vi "get_image.vi"(8 "error in":errorcluster, 9 "height":i32=512, 10 "width":i32=240) -> (0 "error out":errorcluster, 1 "data":u16[][](array[numeric]), 2 "获取单帧图像返回值":i32, 3 "Image":T1(plugin-control), 4 "Intensity Graph":u16[][](graph))   [LabVIEW 2016]
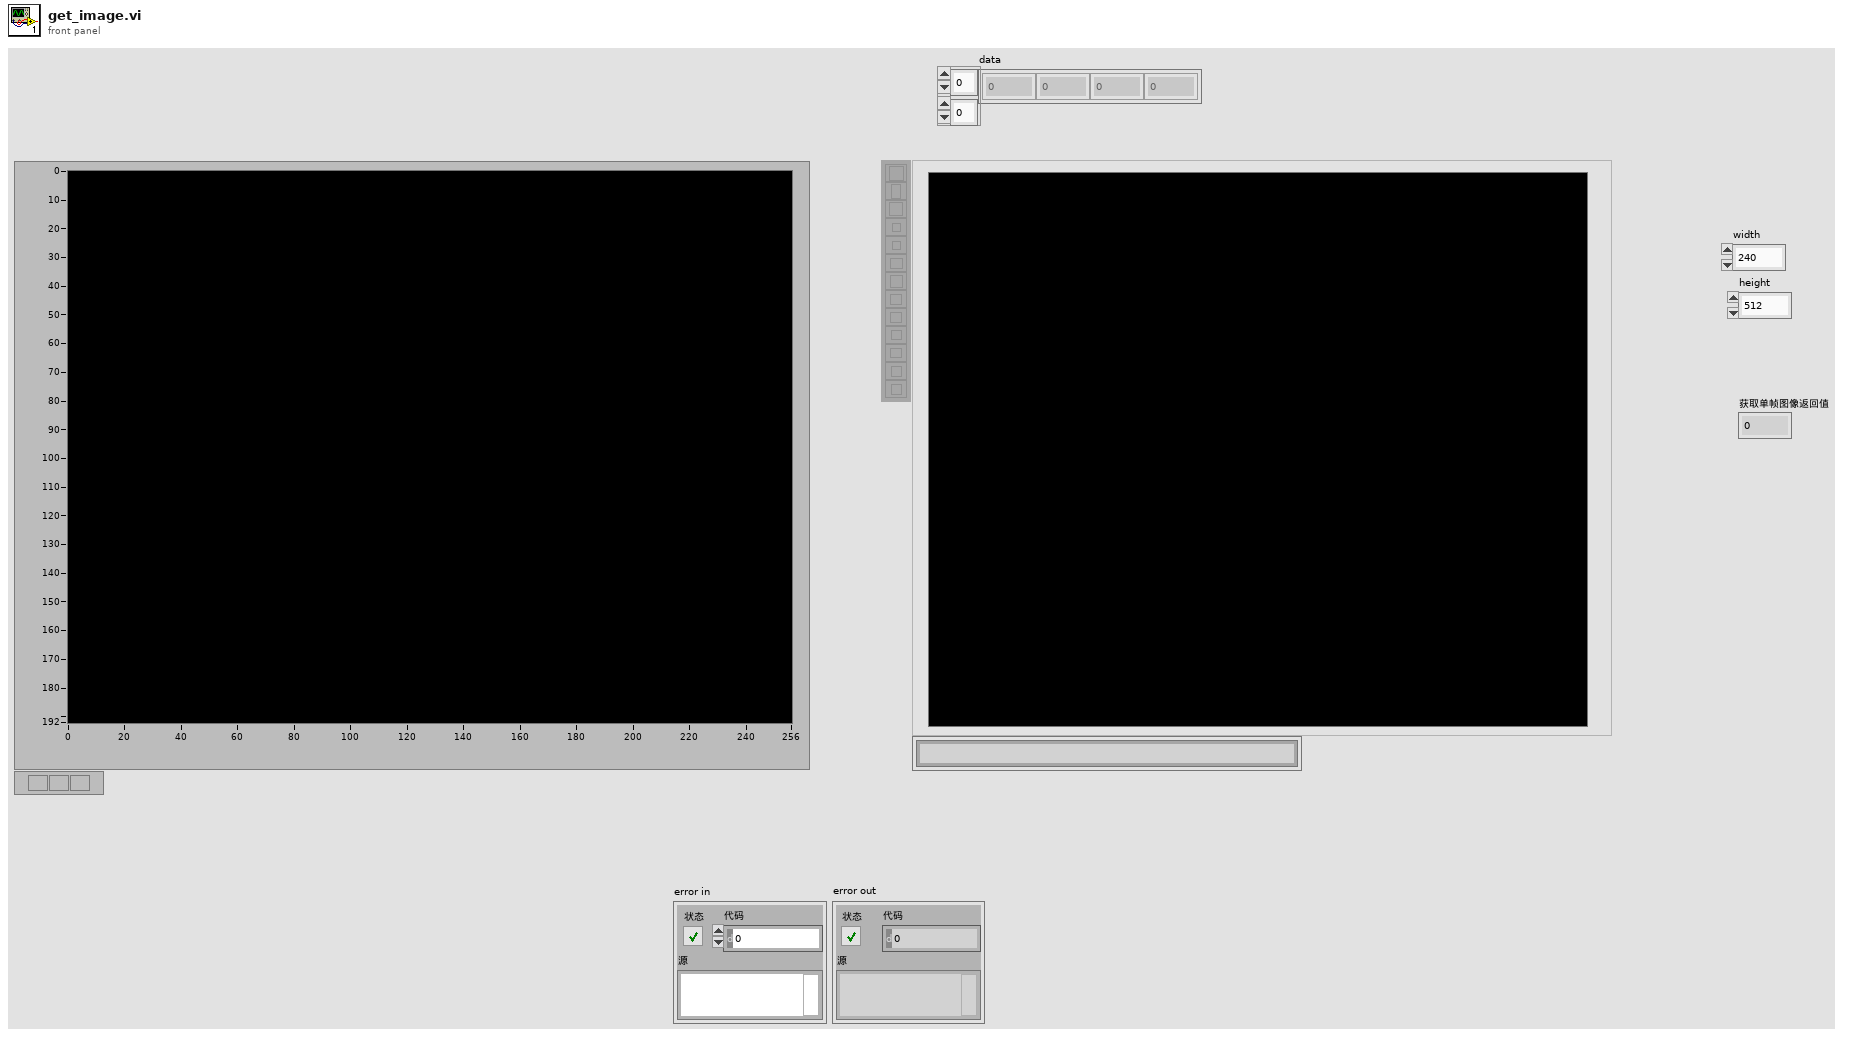
[diagram p1: front panel]
types:
  T1 = typedef "IMAQ Image.ctl" = refnum<image>
  T2 = typedef "Image Type" = u32
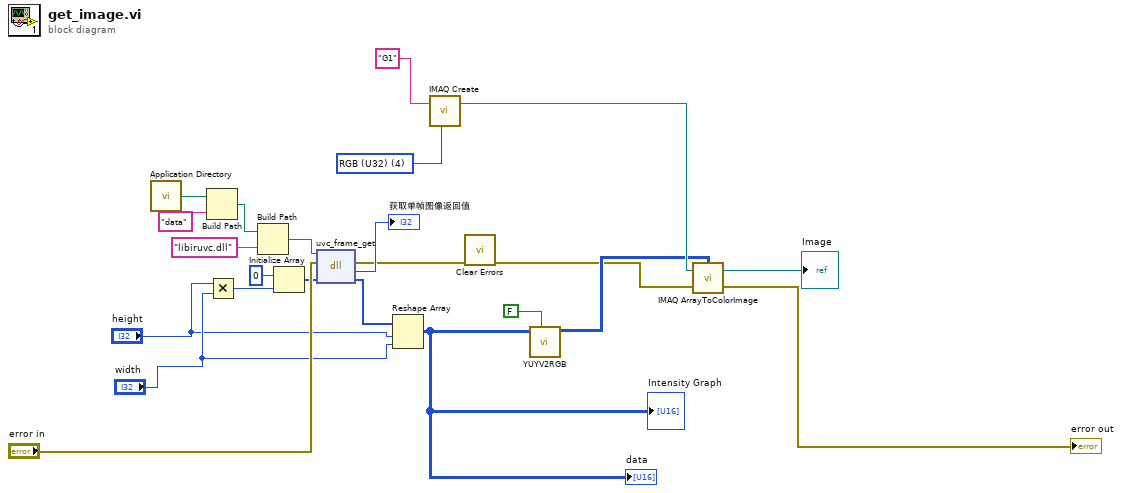
[diagram p0: block diagram]
diagram:
  w23 = T2 4 items=["Grayscale (U8)", "Grayscale (I16)", "Grayscale (SGL)", "Complex (CSG)", "RGB (U32)", "HSL (U32)", "RGB (U64)", "Grayscale (U16)"] ("Image Type")
  n1 = call <vilib>:"Application Directory.vi"() -> ("Application Directory"=w11:path)
  n2 = Build Path(base path=w11, name or relative path="data") -> (appended path=w9:path)
  n3 = Multiply(x="height", y="width") -> (x*y=w14:i32)
  n4 = Build Path(base path=w9, name or relative path="libiruvc.dll") -> (appended path=w15:path)
  n5 = Initialize Array(u16 0, w14) -> (w12:u16[])
  n6 = dll-call lib="D:/libiruvc_0.3.3/windows/x64/dll/libiruvc.dll" fn="uvc_frame_get"(path in=w15, error in="error in", "data"=w12) -> (error out=w6:errorcluster, "return type"=→"获取单帧图像返回值":i32, "data"=w2:u16[])  [unwired: 1 in, 1 out]
  n7 = Reshape Array(w2, "height", "width") -> (w1:u16[][])
  "Intensity Graph" <- w1
  "data" <- w1
  n8 = call "IMAQ Create"("Image Name"="G1", "Image Type"=w23) -> ("New Image"=w21:T1)  [unwired: 3 in, 1 out]
  n9 = call <vilib>:"Clear Errors.vi"("error in (no error)"=w6) -> ("error out"=w5:errorcluster)  [unwired: 5 in, 1 out]
  n10 = call "YUYV2RGB.vi"("1D"=FALSE, "inputArray"=w1) -> ("output array"=w18:u32[][])  [unwired: 9 in]
  n11 = call "IMAQ ArrayToColorImage"("Image Pixels (U32)"=w18, "Image"=w21, "error in (no error)"=w5) -> ("Image Out"=→"Image":T1, "error out"=→"error out":errorcluster)  [unwired: 2 in]
